vi "Query.vi"(8 "error in (no error)":errorcluster, 11 "Ultrasonic Sensor in":refnum<class "Ultrasonic Sensor.lvclass">) -> (0 "error out":errorcluster, 2 "Message":string, 3 "Ultrasonic Sensor out":refnum<class "Ultrasonic Sensor.lvclass">)   [LabVIEW 2021, in "Ultrasonic Sensor.lvclass"]
uses:
  Ultrasonic Sensor.lvclass
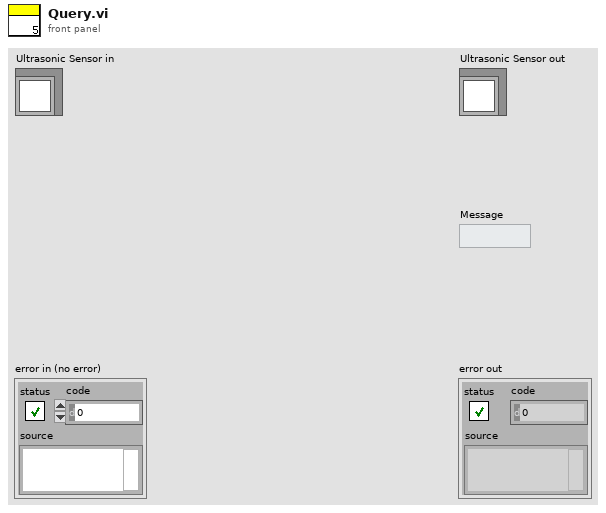
[diagram p1: front panel]
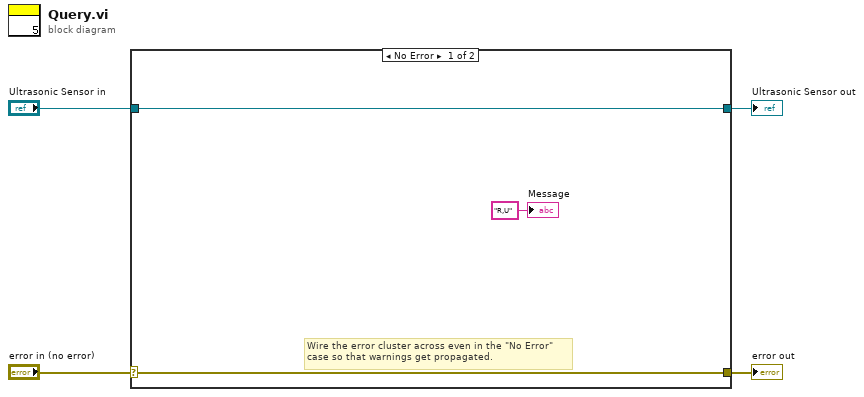
[diagram p0: block diagram]
diagram:
  n1 = case shown="No Error" "error in (no error)" {
    selector: "error in (no error)" -> [w6 w9]
    tunnel: [w6 w9] -> w3
    tunnel: [w7 w8] -> w1
    tunnel: "Ultrasonic Sensor in" -> [w7 w8]
    frame No Error {
      # "Wire the error cluster across even in the \"No Error\"\ncase so that warnings get propagated."
      "Message" <- "R,U" ("Message")
    }
    frame Error {
    }
  }
  "error out" <- w3
  "Ultrasonic Sensor out" <- w1
